vi "Periodic Tasks.vi"(8 "error in":errorcluster) -> ()   [LabVIEW 2017]
doc: "This VI runs in parallel to other tasks. It can contain as many user-defined periodic loops as you need. These can carry out PID or other sorts of timed response."
uses:
  <vilib>/Rock Robotics/WPI/ThirdParty/Phoenix-LabVIEW/Motor Controller/Get/CTRE_Phoenix_MotorController_GetSelectedSensorData.vi
panel:
  in  "Reset":bool
  out "Right Acceleration":dbl(graph)
  out "Left Acceleration":dbl(graph)
  out "Right Position":i32(graph)
  out "Right Velocity":i32(graph)
  out "Left Position":i32(graph)
  out "Left Velocity":i32(graph)
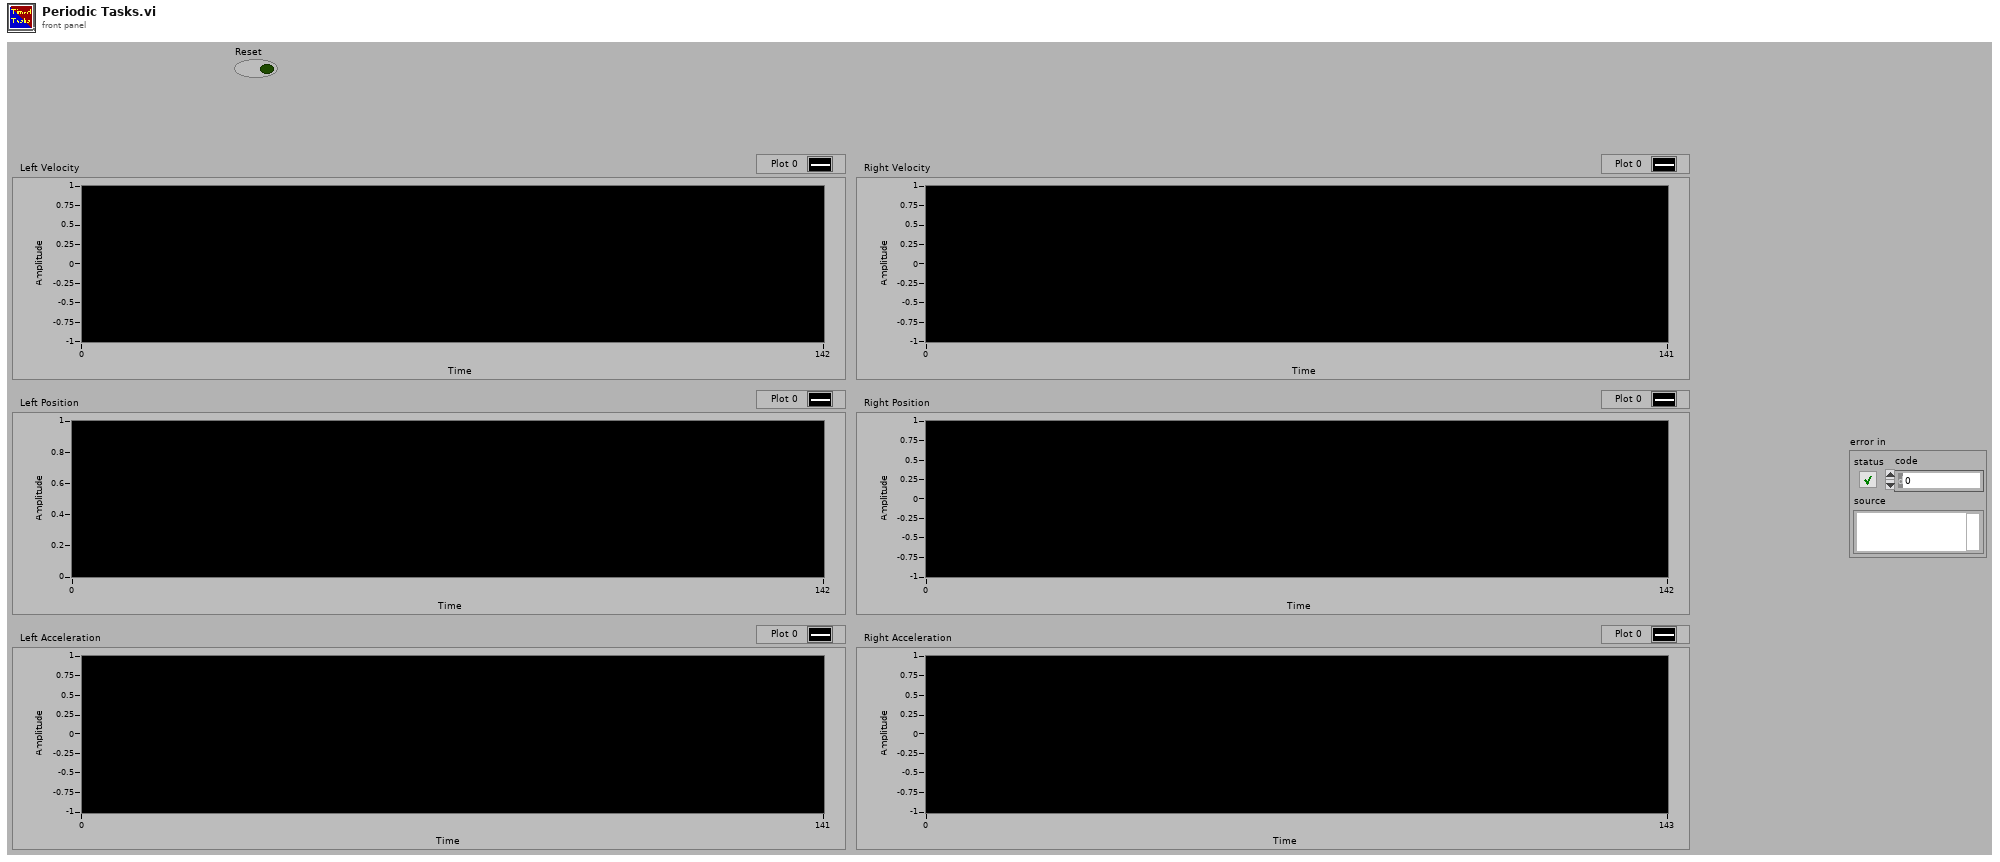
[diagram p1: front panel]
types:
  T1 = typedef "WPI_MotorControlDeviceRef.ctl" = cluster{"DeviceStatus":errorcluster, "Type":T2, "PWM":cluster{"PWM Channel":T3, "DeadBand":T4}, "CAN":cluster{"Device Number":u8, "SetOutput VI Ref":variant, "GetOutput VI Ref":variant, "Enable VI Ref":variant, "Disable VI Ref":variant, "Data":variant}, "Invert":bool, "DIO PWM":cluster{"PWM \"Enable\" Channel":T3, "DIOChannel":T5, "PWM Rate":dbl}}
  T2 = typedef "WPI_MotorControlType.ctl" = enum16{"PWM", "CAN", "DIO PWM"}
  T3 = typedef "FPGA_DIOPWMChannel.ctl" = enum8{"PWM 0", "PWM 1", "PWM 2", "PWM 3", "PWM 4", "PWM 5", "PWM 6", "PWM 7", "PWM 8", "PWM 9", "PWM MXP 0", "PWM MXP 1", "PWM MXP 2", "PWM MXP 3", "PWM MXP 4", "PWM MXP 5", "PWM MXP 6", "PWM MXP 7", "PWM MXP 8", "PWM MXP 9", "Invalid"}
  T4 = typedef "WPI_PWMDeadband.ctl" = cluster{"Name":string, "maxPositivePwm":i32, "minPositivePwm":i32, "centerPwm":i32, "maxNegativePwm":i32, "minNegativePwm":i32, "angularRange":u16}
  T5 = typedef "FPGA_DIOChannel.ctl" = enum8{"DIO 0", "DIO 1", "DIO 2", "DIO 3", "DIO 4", "DIO 5", "DIO 6", "DIO 7", "DIO 8", "DIO 9", "DIO MXP 0", "DIO MXP 1", "DIO MXP 2", "DIO MXP 3", "DIO MXP 4", "DIO MXP 5", "DIO MXP 6", "DIO MXP 7", "DIO MXP 8", "DIO MXP 9", "DIO MXP 10", "DIO MXP 11", "DIO MXP 12", "DIO MXP 13", "DIO MXP 14", "DIO MXP 15", "SPI Port CS1", "SPI Port CS2", "SPI Port CS3", "SPI Port MISO", "SPI Port MOSI", "Invalid"}
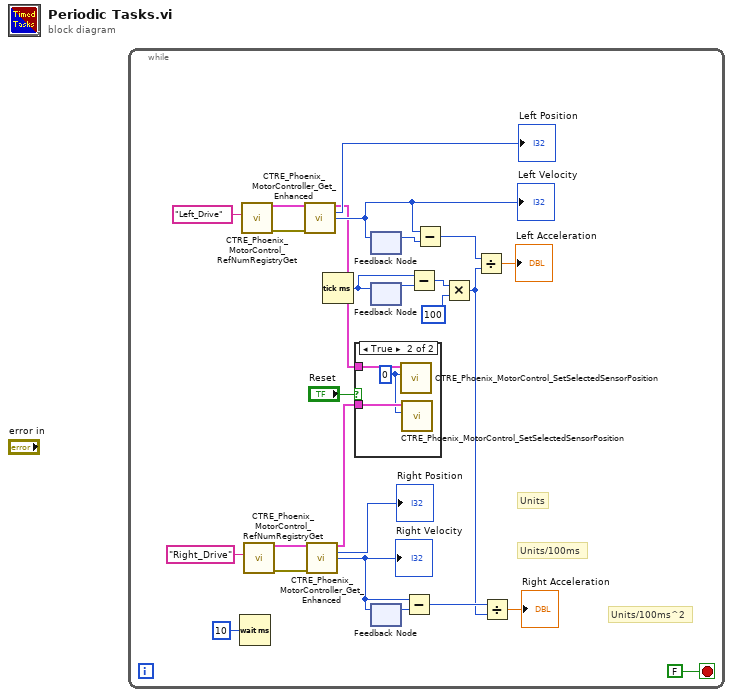
[diagram p0: block diagram]
diagram:
  n1 = while {
    stop <- FALSE stop-if-true
    # "Units/100ms^2"
    # "Units/100ms"
    # "Units"
    n2 = Wait (ms)(milliseconds to wait=u32 10) -> ()  [unwired: 1 out]
    n3 = call <vilib>:"CTRE_Phoenix_MotorControl_RefNumRegistryGet.vi"("refnum name"="Left_Drive") -> ("error out"=w24:errorcluster, "PhoenixMotorControlDevRef"=w25:T1)  [unwired: 9 in]
    n4 = call <vilib>:"CTRE_Phoenix_MotorControl_RefNumRegistryGet.vi"("refnum name"="Right_Drive") -> ("error out"=w20:errorcluster, "PhoenixMotorControlDevRef"=w21:T1)  [unwired: 9 in]
    n5 = call-poly <vilib>:"CTRE_Phoenix_MotorController_Get_Enhanced.vi"("PhoenixMotorControlDevRef"=w25, "error in"=w24) -> ("PhoenixMotorControlDevRef"=w5:T1, "Position (Raw Sensor Units)"=→"Left Position":i32, "Velocity (Raw Sensor Units per 100 ms)"=w17:i32)  [unwired: 10 in, 1 out]
    "Left Velocity" <- w17
    n6 = call-poly <vilib>:"CTRE_Phoenix_MotorController_Get_Enhanced.vi"("PhoenixMotorControlDevRef"=w21, "error in"=w20) -> ("PhoenixMotorControlDevRef"=w4:T1, "Position (Raw Sensor Units)"=→"Right Position":i32, "Velocity (Raw Sensor Units per 100 ms)"=w6:i32)  [unwired: 10 in, 1 out]
    "Right Velocity" <- w6
    n7 = Tick Count (ms)() -> (millisecond timer value=w15:u32)
    n8 = case shown="True" "Reset" {
      tunnel: w5 -> [_ w29]
      tunnel: w4 -> [_ w28]
      frame False {
      }
      frame True {
        w27 = 0 ("New Sensor Position")
        n9 = call <vilib>:"CTRE_Phoenix_MotorControl_SetSelectedSensorPosition.vi"("New Sensor Position"=w27, "PhoenixMotorControlDevRef"=w29) -> ()  [unwired: 8 in, 2 out]
        n10 = call <vilib>:"CTRE_Phoenix_MotorControl_SetSelectedSensorPosition.vi"("New Sensor Position"=w27, "PhoenixMotorControlDevRef"=w28) -> ()  [unwired: 8 in, 2 out]
      }
    }
    n11 = feedback #1() -> (w18:i32)  [unwired: 1 in]
    n12 = feedback-in #1(w17) -> ()
    n13 = feedback #2() -> (w16:u32)  [unwired: 1 in]
    n14 = feedback-in #2(w15) -> ()
    n15 = feedback #3() -> (w10:i32)  [unwired: 1 in]
    n16 = feedback-in #3(w6) -> ()
    n17 = Subtract(x=w6, y=w10) -> (x-y=w9:i32)
    n18 = Subtract(x=w15, y=w16) -> (x-y=w14:u32)
    n19 = Subtract(x=w17, y=w18) -> (x-y=w12:i32)
    n20 = Multiply(x=w14, y=u32 100) -> (x*y=w7:u32)
    n21 = Divide(x=w12, y=w7) -> (x/y=→"Left Acceleration":dbl)
    n22 = Divide(x=w9, y=w7) -> (x/y=→"Right Acceleration":dbl)
  }
